vi "GlobalFileName.vi"() -> ()   [LabVIEW 2022 SP3]
panel:
  out "String":string
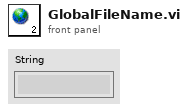
[diagram p1: front panel]
diagram:
